vi "Convectron.vi"(3 "Index":i32[](array[numeric])=[56], 4 "Voltage":u32[](array[numeric])=[3, 3, 3, 1, 2, 3, 3, 3, 5003, 5003, 5003, 5006, 5001, 5004, 5003, 0, 5, 3, 1, 5, 3, 4, 3, 3, 3, 5004, 6, 5003, 4, 5, 5, 5, 4, 1004, 1003, 6, 4, 4, 7, 4, 5, 4, 3, 2, 3, 5, 1, 3, 3, 1, 3, 1, 3, 2, 7, 0, 3000, 9, 0, 0, 0, 0, 8, 7], 5 "Scale":dbl[](array[numeric])=[0.012, 0.06, 0.30000000000000004, 0.02, 0.08, 0.06, 0.30000000000000004, 0.30000000000000004, 1000.6, 1000.6, 1000.6, 1001.2, 1000.2, 1000.8000000000001, 1000.6, 0.0, 1.0, 0.06, 0.2, 0.1, 60.00000000000001, 4.0, 3.0, 18.0, 0.30000000000000004, 0.0799999999999983, 0.6000000000000001, 0.060000000000002274, 4.0, 5.0, 5.0, 5.0, 1.3332, 1.5, 1.125, 0.0006000000000000001, 0.4, 0.4, 0.7000000000000001, 0.4, 1.0, 0.8, 0.06, 0.04, 0.6000000000000001, 0.5, 0.4, 0.30000000000000004, 0.6000000000000001, 0.02, 0.06, 0.2, 1.2000000000000002, 0.4, 0.7000000000000001, nan, 300.0, 0.9, nan, nan, nan, nan, 450.84, 450.735] format="%.2f") -> (1 "Scale out":dbl[](array[numeric])=[0.012, 0.06, 0.30000000000000004, 0.02, 0.08, 0.06, 0.30000000000000004, 0.30000000000000004, 1000.6, 1000.6, 1000.6, 1001.2, 1000.2, 1000.8000000000001, 1000.6, 0.0, 1.0, 0.06, 0.2, 0.1, 60.00000000000001, 4.0, 3.0, 18.0, 0.30000000000000004, 0.0799999999999983, 0.6000000000000001, 0.060000000000002274, 4.0, 5.0, 5.0, 5.0, 1.3332, 1.5, 1.125, 0.0006000000000000001, 0.4, 0.4, 0.7000000000000001, 0.4, 1.0, 0.8, 0.06, 0.04, 0.6000000000000001, 0.5, 0.4, 0.30000000000000004, 0.6000000000000001, 0.02, 0.06, 0.2, 1.2000000000000002, 0.4, 0.7000000000000001, nan, 2.3733227222273405, 0.9, nan, nan, nan, nan, 450.84, 450.735] format="%.2f")   [LabVIEW 2011]
uses:
  <vilib>/Analysis/NI_AALBase.lvlib
panel:
  in  "High":dbl[](array[numeric])=[361816005.34, -413297822.47, 196553071.14, -49816080.153, 7097033.1066, -538887.77795, 17039.048857, 0.0] format="%.10e"
  in  "Mid":dbl[](array[numeric])=[0.10311295434, -0.023222519703, 0.072294948746, -0.3986063871, 0.074382021328, -0.0068656810268] format="%.10e"
  in  "Low":dbl[](array[numeric])=[-0.033114122859, 0.091225738708, -0.10902742405, 0.3431398142, -0.22851221698, 0.094706717562, -0.020686516159, 0.0020209521035] format="%.10e"
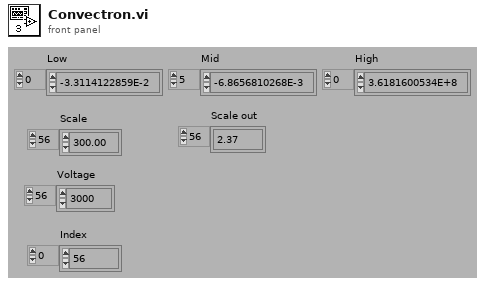
[diagram p1: front panel]
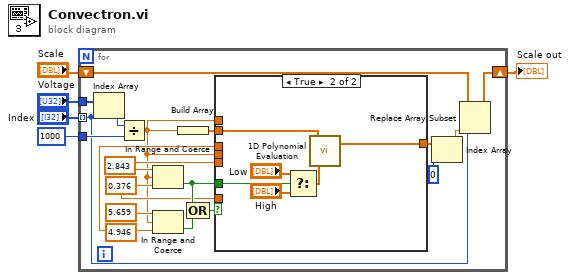
[diagram p0: block diagram]
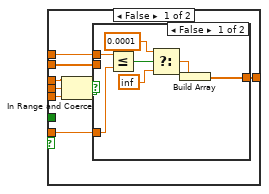
[diagram p2: hidden frame]
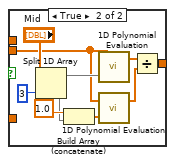
[diagram p3: hidden frame]
diagram:
  n1 = for {
    shift-right: [w14] -> w4
    shift-left: "Scale" -> [w13]
    tunnel: "Index" -> [w9] mode=indexing
    tunnel: "Voltage" -> [w12]
    tunnel: 1000 -> [w10]
    w22 = 4.946
    w7 = 2.843
    w8 = 0.376
    n2 = Index Array(array=w12, index=w9) -> (element=w11:u32)
    n3 = Divide(x=w11, y=w10) -> (x/y=w6:dbl)
    n4 = In Range and Coerce(upper limit=w7, x=w6, lower limit=w8) -> (In Range?=w18:bool)  [unwired: 1 out]
    n5 = In Range and Coerce(upper limit=5.659, x=w6, lower limit=w22) -> (In Range?=w21:bool)  [unwired: 1 out]
    n6 = Build Array(w6) -> (w19:dbl[])
    n7 = Compound Arithmetic op=OR(w18, w21) -> (w20:bool)
    n8 = case shown="True" w20 {
      tunnel: w19 -> [w27 w54]
      tunnel: w18 -> [_ w53]
      tunnel: [w26 w49] -> w17
      tunnel: w6 -> [w31 _]
      tunnel: w22 -> [w30 _]
      tunnel: w7 -> [w29 _]
      tunnel: w6 -> [w25 _]
      tunnel: w8 -> [w24 _]
      frame False {
        n9 = In Range and Coerce(upper limit=w30, x=w31, lower limit=w29) -> (In Range?=w28:bool)  [unwired: 1 out]
        n10 = case shown="False" w28 {
          tunnel: w27 -> [_ w42]
          tunnel: [w38 w39] -> w26
          tunnel: w25 -> [w37 _]
          tunnel: w24 -> [w36 _]
          frame False {
            n11 = Less Or Equal?(x=w37, y=w36) -> (x <= y?=w35:bool)
            n12 = Select(t=0.0001, s=w35, f=inf) -> (s? t:f=w33:dbl)
            n13 = Build Array(w33) -> (w38:dbl[])
          }
          frame True {
            n14 = Split 1D Array(array="Mid", index=3) -> (first subarray=w44:dbl[], second subarray=w47:dbl[])
            n15 = Build Array (concatenate)(1.0, w47) -> (w43:dbl[])
            n16 = call <vilib>:"1D Polynomial Evaluation.vi"("Coefficients: a"=w44, "X"=w42) -> ("Y"=w41:dbl[])  [unwired: 1 out]
            n17 = call <vilib>:"1D Polynomial Evaluation.vi"("Coefficients: a"=w43, "X"=w42) -> ("Y"=w40:dbl[])  [unwired: 1 out]
            n18 = Divide(x=w41, y=w40) -> (x/y=w39:dbl[])
          }
        }
      }
      frame True {
        n19 = Select(t="Low", s=w53, f="High") -> (s? t:f=w50:dbl[])
        n20 = call <vilib>:"1D Polynomial Evaluation.vi"("Coefficients: a"=w50, "X"=w54) -> ("Y"=w49:dbl[])  [unwired: 1 out]
      }
    }
    n21 = Index Array(array=w17, index=0) -> (element=w15:dbl)
    n22 = Replace Array Subset(array=w13, new element=w15, index=w9) -> (w14:dbl[])
  }
  "Scale out" <- w4
